vi "Reg Scan Counter.vi"(7 "Action":T1, 11 "# of Steps":i32) -> (1 "Scan Done?":bool, 3 "Current Step":i32)   [LabVIEW 2016]
uses:
  Reg Counter Action.ctl
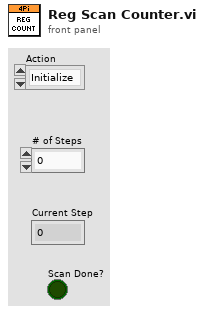
[diagram p1: front panel]
types:
  T1 = typedef "Reg Counter Action.ctl" = enum16{"Initialize", "Update Count"}
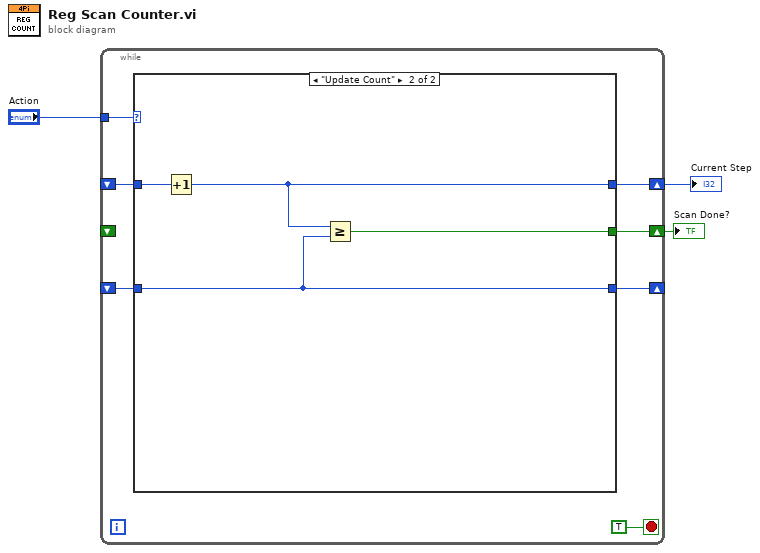
[diagram p0: block diagram]
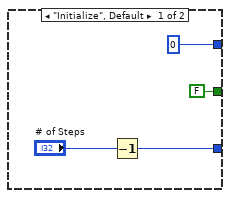
[diagram p2: hidden frame]
diagram:
  n1 = while {
    tunnel: "Action" -> [w10]
    shift-right: [w8] -> w2
    shift-left: _ -> [w7]
    shift-right: [w6] -> _
    shift-left: _ -> [w5]
    shift-right: [w4] -> w1
    shift-left: _ -> [_]
    stop <- TRUE stop-if-true
    n2 = case shown="\"Update Count\"" w10 {
      tunnel: [0 w17] -> w8
      tunnel: w7 -> [_ w18]
      tunnel: [w11 w16] -> w6
      tunnel: w5 -> [_ w16]
      tunnel: [FALSE w15] -> w4
      frame "Initialize", Default {
        n3 = Decrement(x="# of Steps") -> (x-1=w11:i32)
      }
      frame "Update Count" {
        n4 = Increment(x=w18) -> (x+1=w17:i32)
        n5 = Greater Or Equal?(x=w17, y=w16) -> (x >= y?=w15:bool)
      }
    }
  }
  "Current Step" <- w2
  "Scan Done?" <- w1
